vi "Stop Core.vi"(10 "final error code":i32, 11 "Flex UI (Actor) in":refnum<class "Flex UI (Actor).lvclass">) -> (3 "Flex UI (Actor) out":refnum<class "Flex UI (Actor).lvclass">)   [LabVIEW 2016, in "Flex UI (Parent Actor).lvlib" / "Flex UI (Actor).lvclass"]
doc: "(<B>Filename</B>: Actor Framework.lvlib:Actor.lvclass:Stop Core.vi)\n\nDefines what the actor does before it stops. Use the <B>final error code</B> input to determine whether the actor shut down in response to an error.\n\nBy default, this method does nothing. A descendant class may override it to define behavior, such as shutting down any processes the actor initiated in its override of the Actor Core method."
uses:
  Flex UI (Actor).lvclass
  <vilib>/East West Architects/Parent Actor Template/_Parent Actor Template.lvclass
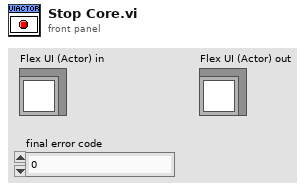
[diagram p1: front panel]
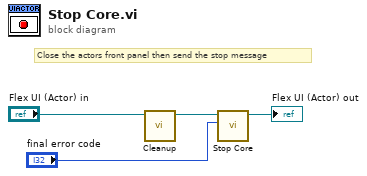
[diagram p0: block diagram]
diagram:
  # "Close the actors front panel then send the stop message"
  n1 = call-dynamic "Cleanup.vi"("Flex UI (Actor) in"="Flex UI (Actor) in") -> ("Flex UI (Actor) out"=w1:refnum<class "Flex UI (Actor).lvclass">)  [unwired: 9 in, 1 out]
  n2 = call-parent "Stop Core.vi"("final error code"="final error code", "_Parent Actor Template in"=w1) -> ("_Parent Actor Template out"=→"Flex UI (Actor) out":refnum<class "Flex UI (Actor).lvclass">)  [unwired: 9 in]
